vi "New Targets Update from JSON.vi"(2 "error in":errorcluster, 3 "Targets Message":T2={"capturedAgoMs"=0, "targets"=[{"x"=0.0, "y"=0.0, "z"=0.0, "theta"=0.0}]}, 4 "Current Time (ms)":dbl) -> (0 "error out":errorcluster, 1 "Targets Update":T1)   [LabVIEW 2016]
uses:
  Targets Message.ctl
  Targets Info.ctl
  Targets Update.ctl
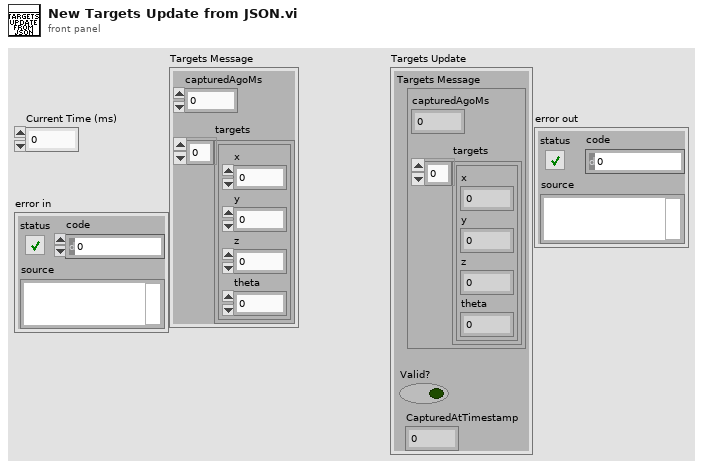
[diagram p1: front panel]
types:
  T1 = typedef "Targets Update.ctl" = cluster{"Valid?":bool, "CapturedAtTimestamp":dbl, "Targets Message":T2}
  T2 = typedef "Targets Message.ctl" = cluster{"capturedAgoMs":i32, "targets":T3[]}
  T3 = typedef "Targets Info.ctl" = cluster{"x":dbl, "y":dbl, "z":dbl, "theta":dbl}
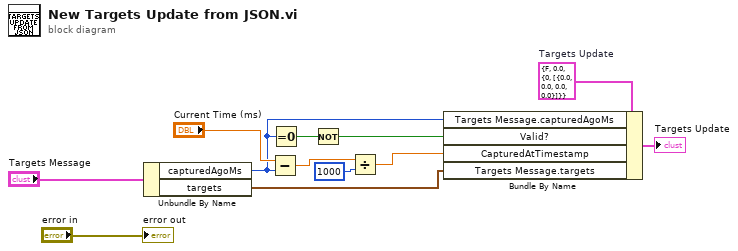
[diagram p0: block diagram]
diagram:
  w4 = T1 {"Valid?"=FALSE, "CapturedAtTimestamp"=0.0, "Targets Message"={"capturedAgoMs"=0, "targets"=[{"x"=0.0, "y"=0.0, "z"=0.0, "theta"=0.0}]}}  # Targets Update
  n1 = Unbundle By Name("Targets Message") -> ("capturedAgoMs"=w3:i32, "targets"=w2:T3[])
  n2 = Subtract(x="Current Time (ms)", y=w3) -> (x-y=w10:dbl)
  n3 = Equal To 0?(x=w3) -> (x = 0?=w12:bool)
  n4 = Not(x=w12) -> (.not. x?=w8:bool)
  n5 = Divide(x=w10, y=1000) -> (x/y=w7:dbl)
  n6 = Bundle By Name(cluster=w4, "Targets Message.capturedAgoMs"=w3, "Valid?"=w8, "CapturedAtTimestamp"=w7, "Targets Message.targets"=w2) -> (→"Targets Update":T1)
  "error out" <- "error in"
